vi "ziGetEventScopeWave.vi"(8 "Error In":errorcluster, 10 "ScopeWave In":T1={"Timestamp (ticks)"=0, "Timestamp Trigger (ticks)"=0, "dt (s)"=0.0, "Channel Enable"=[], "Channel Input"=[], "Trigger Enable"=0, "Trigger Input"=0, "Channel BW Limit"=[], "Channel Math"=[], "Channel Scaling"=[], "Sequence Number"=0, "Segment Number"=0, "Block Number"=0, "Data Transfer Mode"=enum."Single Transfer", "Block Marker"=enum."None", "Flags"=0, "Sample Format"=enum."Int32 Interleaved", "Sample Count"=0, "Channel Offset"=[], "Data Int16"=[], "Data Int32"=[], "Data Float"=[], "Total Samples"=0} {"dt (s)" format="%#_6p"}, 11 "Handle In":T2 {"Handle" format="0x%08x"; "Conn" format="0x%08x"}) -> (0 "Error Out":errorcluster, 2 "ScopeWave Out":T1={"Timestamp (ticks)"=0, "Timestamp Trigger (ticks)"=0, "dt (s)"=0.0, "Channel Enable"=[], "Channel Input"=[], "Trigger Enable"=0, "Trigger Input"=0, "Channel BW Limit"=[], "Channel Math"=[], "Channel Scaling"=[], "Sequence Number"=0, "Segment Number"=0, "Block Number"=0, "Data Transfer Mode"=enum."Single Transfer", "Block Marker"=enum."None", "Flags"=0, "Sample Format"=enum."Int32 Interleaved", "Sample Count"=0, "Channel Offset"=[], "Data Int16"=[], "Data Int32"=[], "Data Float"=[], "Total Samples"=0} {"dt (s)" format="%#_6p"}, 3 "Handle Out":T2 {"Handle" format="0x%08x"; "Conn" format="0x%08x"})   [LabVIEW 2009, in "Zurich Instruments LabOne.lvlib"]
doc: "This vi retives scope data. The data may be formatted differently, depending on settings of the scope. See the description of the structure members for details."
uses:
  <instrlib>/Zurich Instruments LabOne/Zurich Instruments LabOne.lvlib
  <instrlib>/Zurich Instruments LabOne/Public/ziTypeHandle.ctl
  <instrlib>/Zurich Instruments LabOne/Public/Data/ziTypeScopeWave.ctl
  <instrlib>/Zurich Instruments LabOne/Private/ziLV64.dll
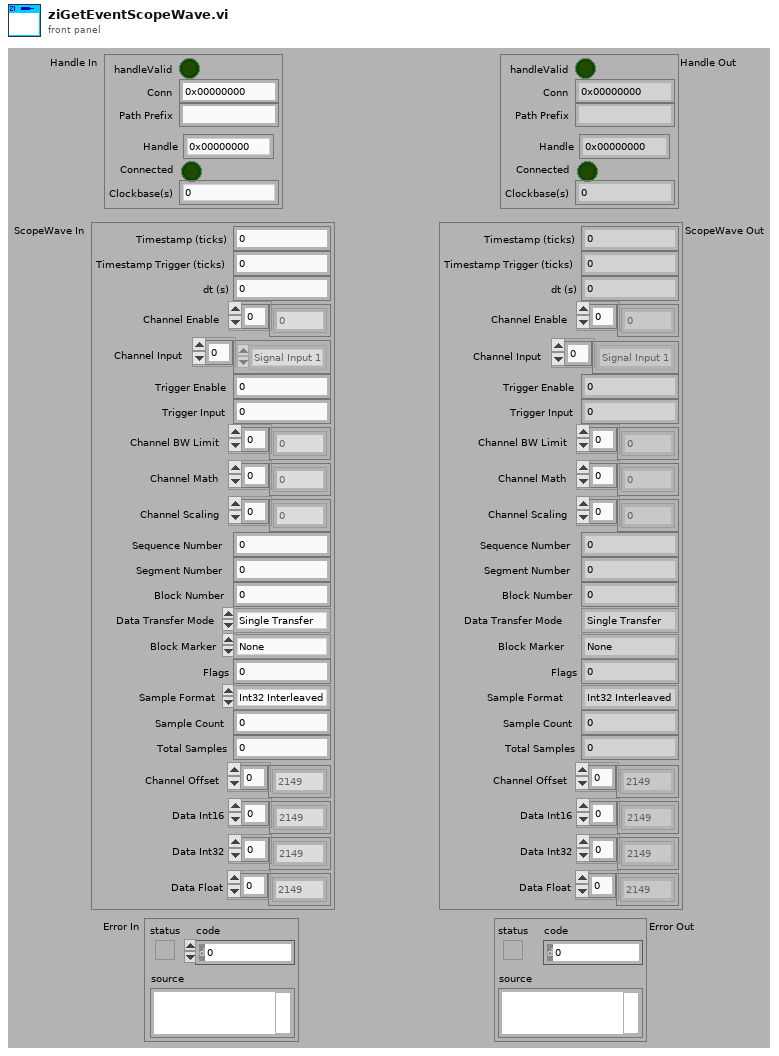
[diagram p1: front panel]
types:
  T1 = typedef "Zurich Instruments LabOne.lvlib/ziTypeScopeWave.ctl" = cluster{"Timestamp (ticks)":u64, "Timestamp Trigger (ticks)":u64, "dt (s)":dbl, "Channel Enable":u8[], "Channel Input":enum8{"Signal Input 1", "Signal Input 2", "Trigger Input 1", "Trigger Input 2", "Aux Output 1", "Aux Output 2", "Aux Output 3", "Aux Output 4", "Aux Input 1", "Aux Input 2"}[], "Trigger Enable":u64, "Trigger Input":u64, "Channel BW Limit":u8[], "Channel Math":u8[], "Channel Scaling":sgl[], "Sequence Number":u32, "Segment Number":u32, "Block Number":u32, "Data Transfer Mode":enum8{"Single Transfer", "Block Transfer", "Continuous Transfer", "FFT Single Transfer"}, "Block Marker":enum8{"None", "End of Block"}, "Flags":u8, "Sample Format":enum8{"Int16", "Int32", "Float32", "reserved", "Int16 Interleaved", "Int32 Interleaved", "Float32 Interleaved"}, "Sample Count":u32, "Channel Offset":dbl[], "Data Int16":i16[], "Data Int32":i32[], "Data Float":sgl[], "Total Samples":u64}
  T2 = typedef "Zurich Instruments LabOne.lvlib/ziTypeHandle.ctl" = cluster{"handleValid":bool, "Conn":u64, "Path Prefix":string, "Handle":u64, "Connected":bool, "Clockbase(s)":dbl}
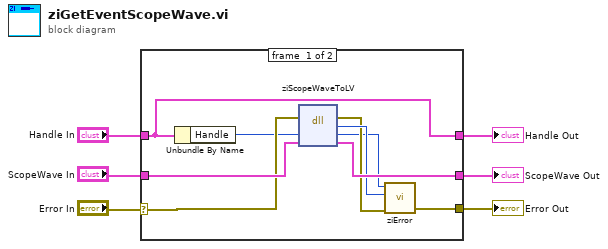
[diagram p0: block diagram]
diagram:
  n1 = case shown="No Error" "Error In" {
    selector: "Error In" -> [w12 w18]
    tunnel: "Handle In" -> [w8 w16]
    tunnel: [w8 w16] -> w5
    tunnel: [w15 w17] -> w4
    tunnel: "ScopeWave In" -> [w14 w17]
    tunnel: [w13 w18] -> w3
    frame #0 {
      n2 = Unbundle By Name(w8) -> ("Handle"=w11:u64)
      n3 = dll-call lib="C:/Program Files/National Instruments/LabVIEW 2009/instr.lib/Zurich Instruments LabOne/Private/ziLV*.*" fn="ziScopeWaveToLV"(error in=w12, "ziEventBuffer"=w11, "ScopeWave"=w14) -> (error out=w9:errorcluster, "return type"=w10:u32, "ziEventBuffer"=w7:u64, "ScopeWave"=w15:T1)  [unwired: 2 in, 1 out]
      n4 = call <instrlib>:"ziError.vi"("Conn"=w7, "ziErrorCode"=w10, "Error In"=w9) -> ("Error Out"=w13:errorcluster)  [unwired: 2 in, 1 out]
    }
    frame #1 {
    }
  }
  "Handle Out" <- w5
  "ScopeWave Out" <- w4
  "Error Out" <- w3
